vi "Init Base Graph 1.vi"(11 "IntensityGraph in":refnum<vi>) -> (3 "Base Graph out":refnum<class "Base Graph.lvclass">)   [LabVIEW 2023]
uses:
  source/Base Graph/Base Graph.lvclass
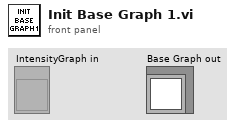
[diagram p1: front panel]
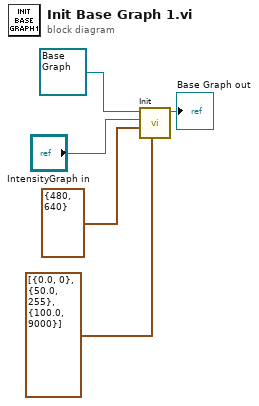
[diagram p0: block diagram]
diagram:
  n1 = call "Init.vi"("Z Scale.Marker Values[]"=cluster{dbl, u32}[] [{0.0, 0}, {50.0, 255}, {100.0, 9000}], "Size"=cluster{"Height":u32, "Width":u32} {"Height"=480, "Width"=640}, "Intensity Graph"="IntensityGraph in", "Base Graph in"=refnum<class "Base Graph.lvclass"> refnum ("Base Graph.lvclass")) -> ("Base Graph out"=→"Base Graph out":refnum<class "Base Graph.lvclass">)  [unwired: 6 in, 1 out]
